vi "Scripting_ConvertNativeBaseClassToSubClass.vi"(0 "BaseClass":refnum<vi>, 1 "NewBaseClass":path=path "C:/Projects/P1G/N1_class/N1.lvclass", 5 "error in (no error)":errorcluster) -> (19 "error out":errorcluster={"status"=TRUE, "code"=1055, "source"="Property Node in Scripting_ConvertBaseClassToSubClass.vi"})   [LabVIEW 2020]
uses:
  <resource>/Framework/Providers/Open_GDS/ClassProviders/Provider_LvNativeClass/Templates/LvNativeTemplateNames.ctl
  <resource>/Framework/Providers/Open_GDS/ClassProviders/Provider_LvNativeClass/ClassWriterNative_class/ClassWriterNative.lvclass
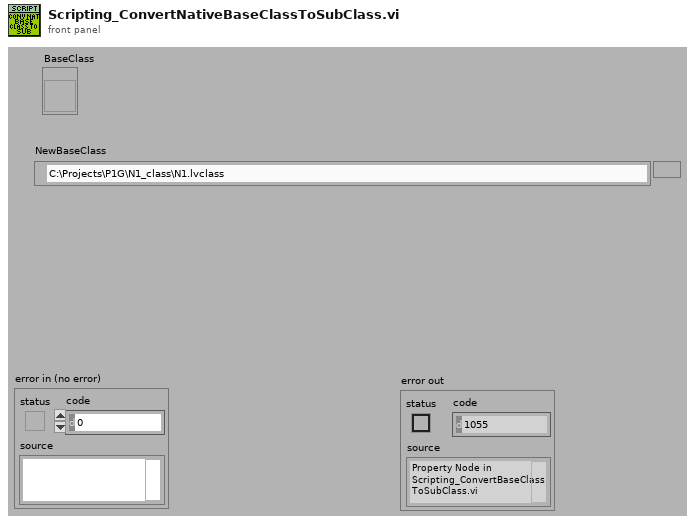
[diagram p1: front panel]
types:
  T1 = cluster{"NewBaseClass":refnum<vi>, "NewBaseCreate ":path, "NewBaseDestroy":path, " BaseClass":refnum<vi>, "BaseCreate ":path, "BaseDestroy":path, "BaseClassName":string, "AllBaseClassFiles":path[], "BaseNewVi":path, "BaseDeleteVi":path, "App":refnum<vi>}
  T2 = typedef "LvNativeTemplateNames.ctl" = enum16{"NativeBaseTemplate", "NativeSubTemplate", "NativeBaseTemplate_4x4x4", "NativeSubTemplate_4x4x4"}
  T3 = typedef "GDSLvCLass_ClassSettingsType.ctl" = cluster{"ClassProviderName":string, "ClassTemplateUsed":string, "ClassTemplateVersion":string, "ClassDescription":string, "PlugIns":T4[], "ConnectorPanePattern":string}
  T4 = typedef "GDSLvClass_PlugIn.ctl" = cluster{"Type":T5, "ID":string, "Version":string, "Path":path, "Name":string, "Data":variant}
  T5 = typedef "GDSLvClass_PlugInTypes.ctl" = enum16{"DesignPattern", "MethodTypes"}
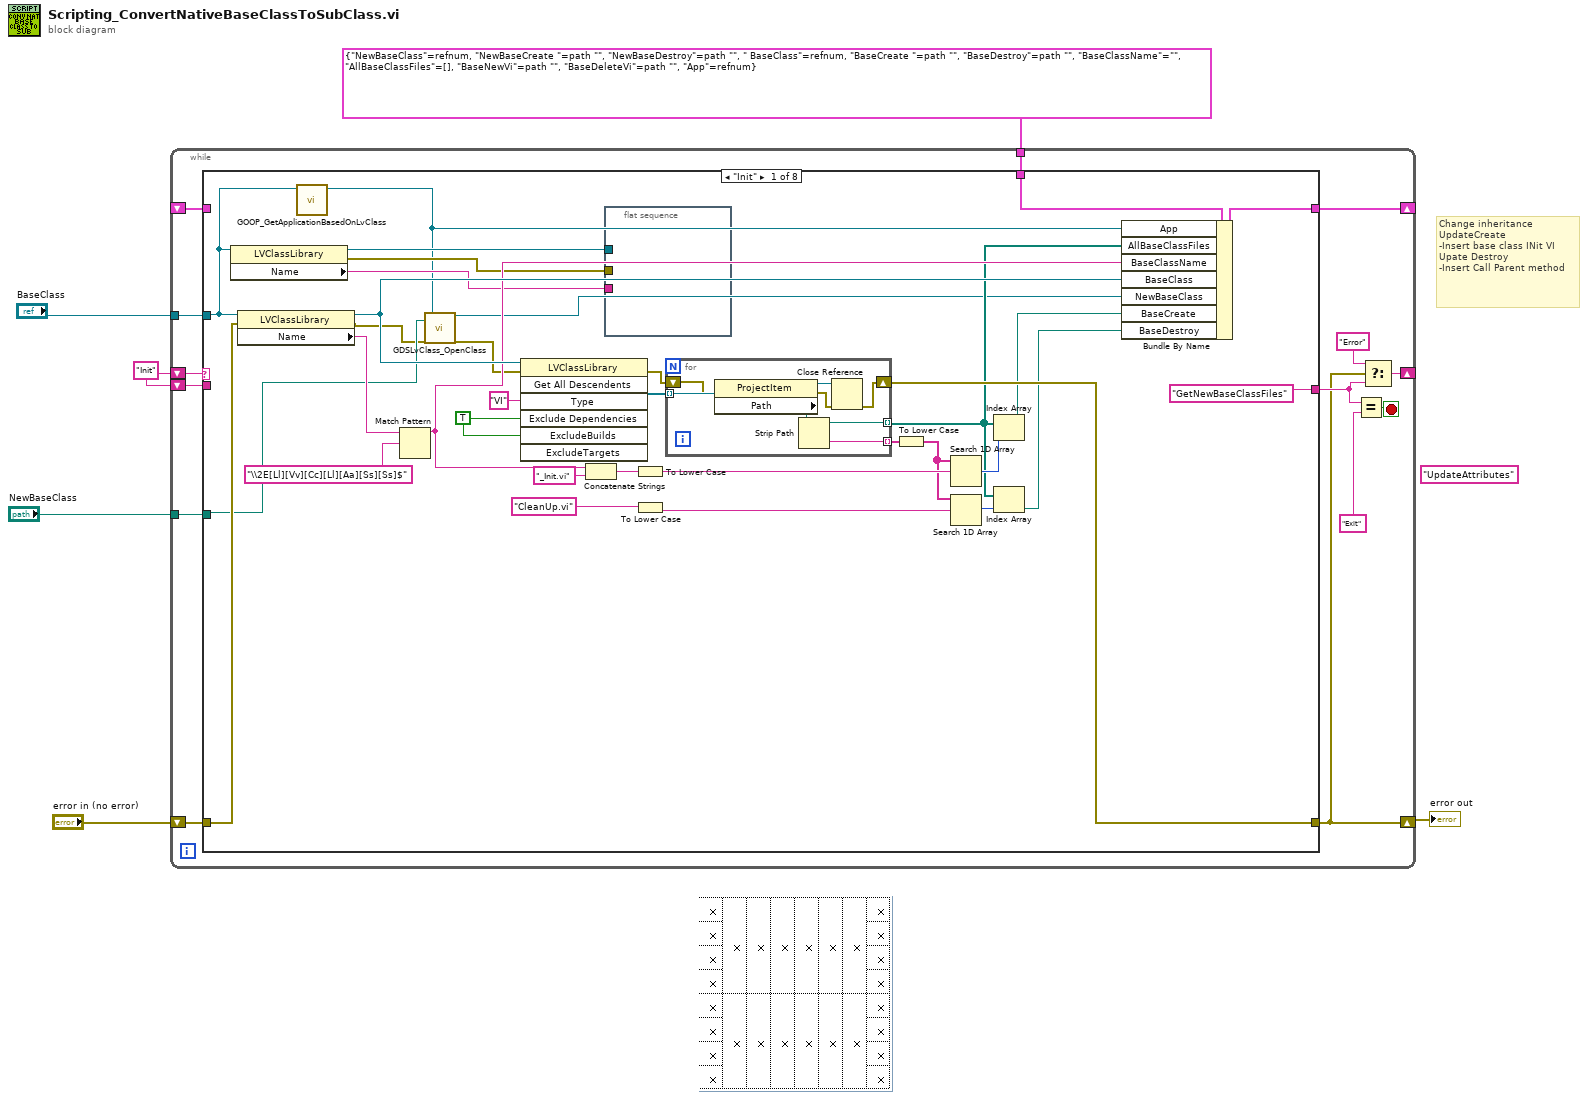
[diagram p0: block diagram]
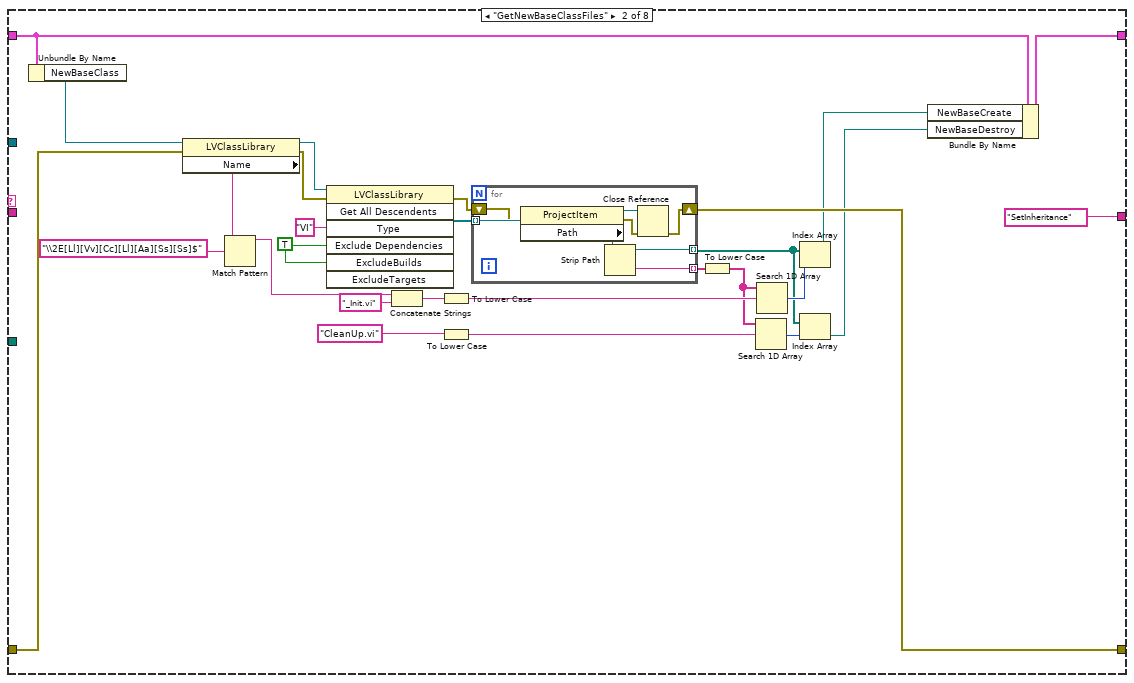
[diagram p2: hidden frame]
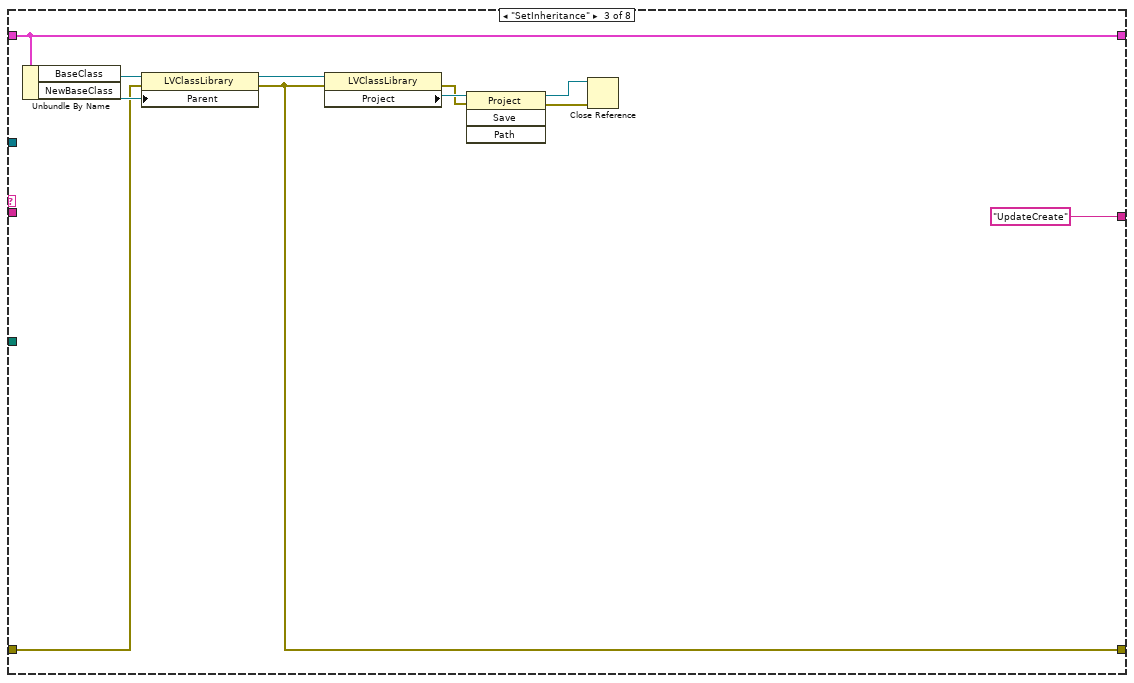
[diagram p3: hidden frame]
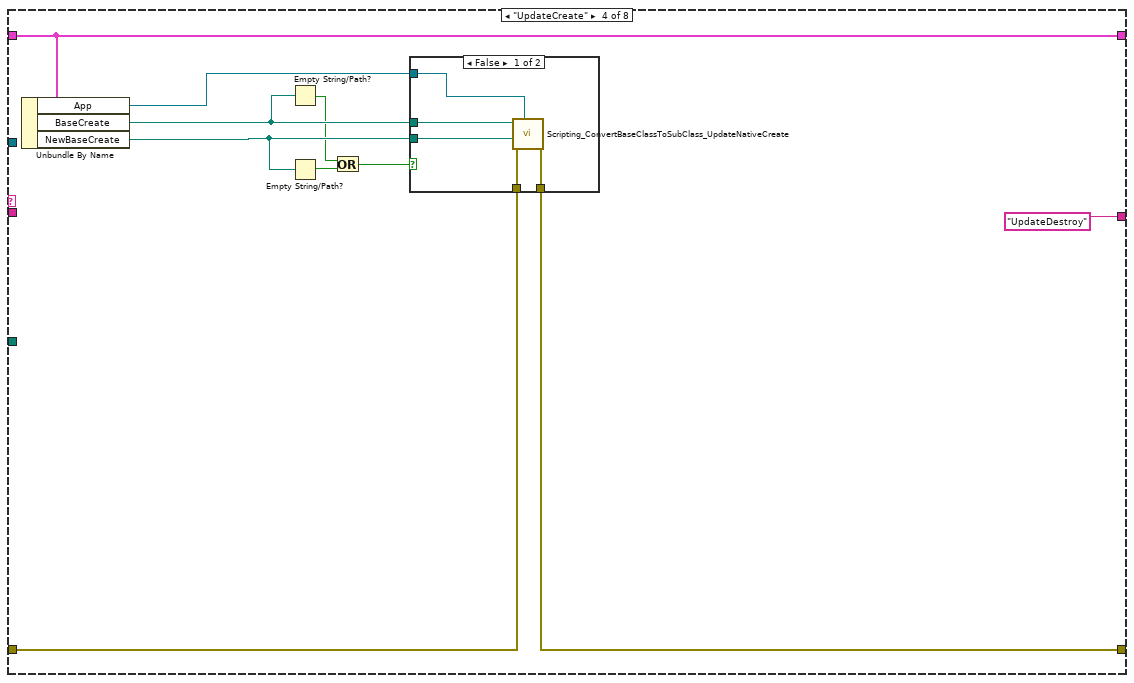
[diagram p4: hidden frame]
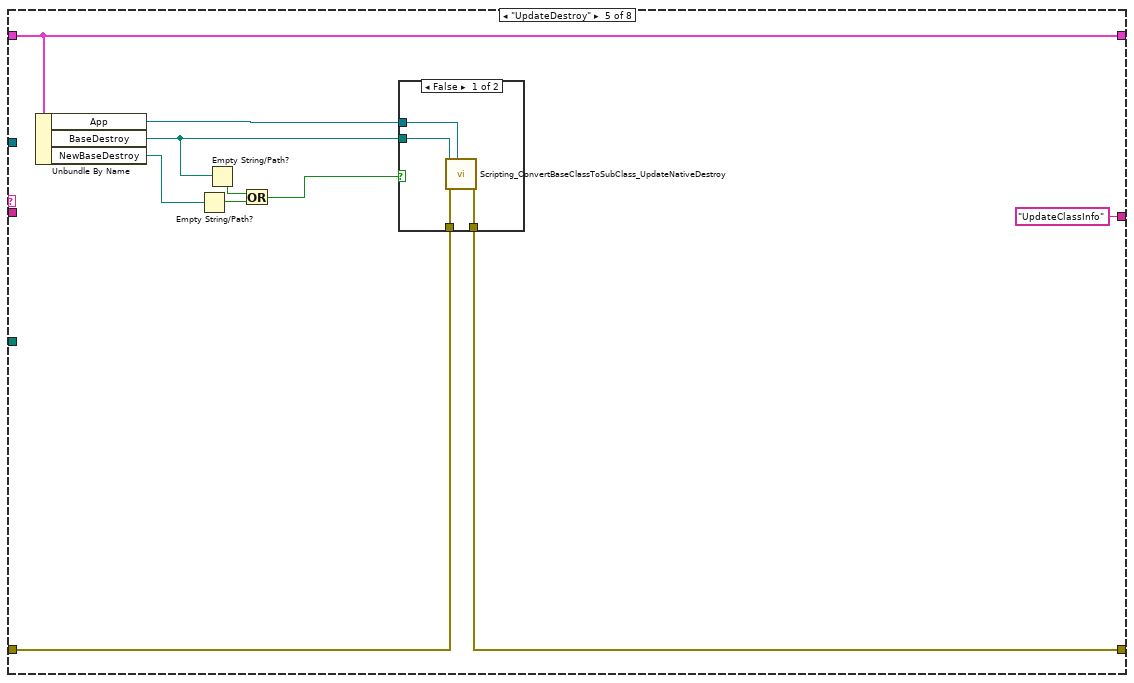
[diagram p6: hidden frame]
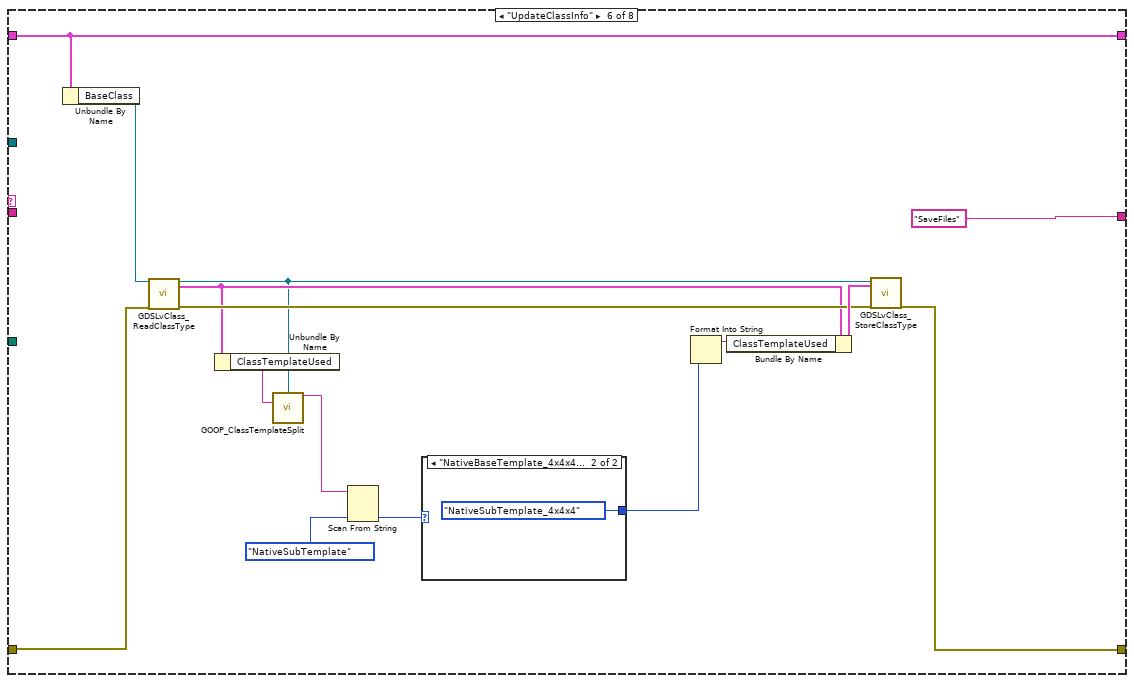
[diagram p8: hidden frame]
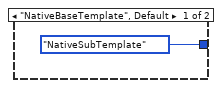
[diagram p9: hidden frame]
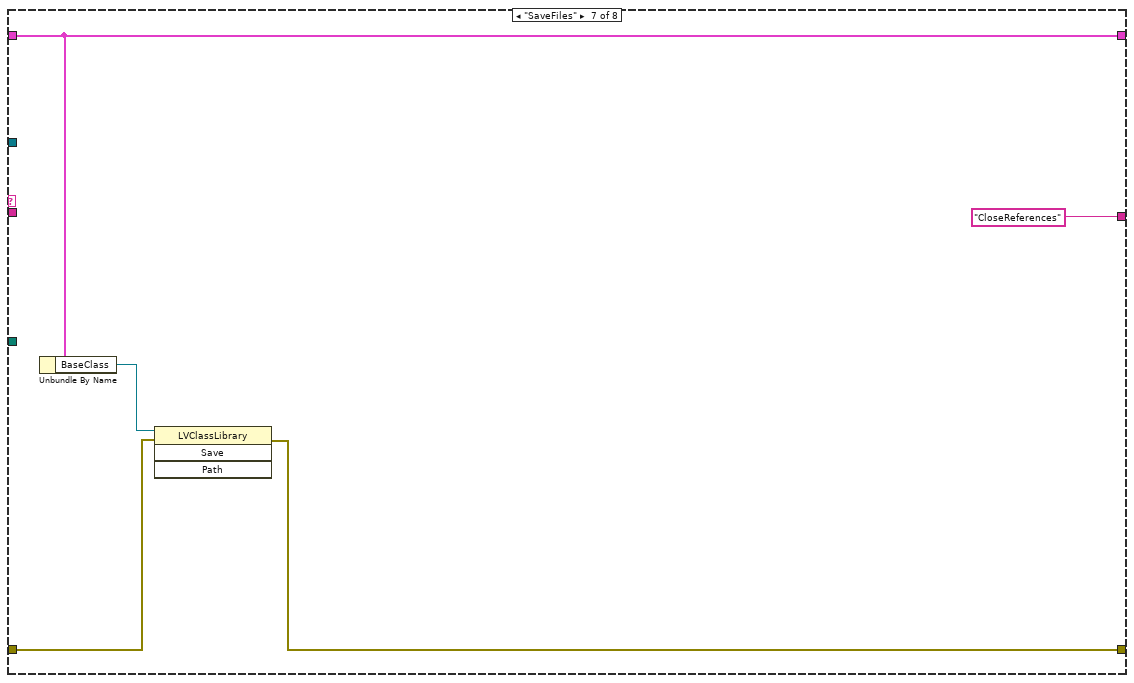
[diagram p10: hidden frame]
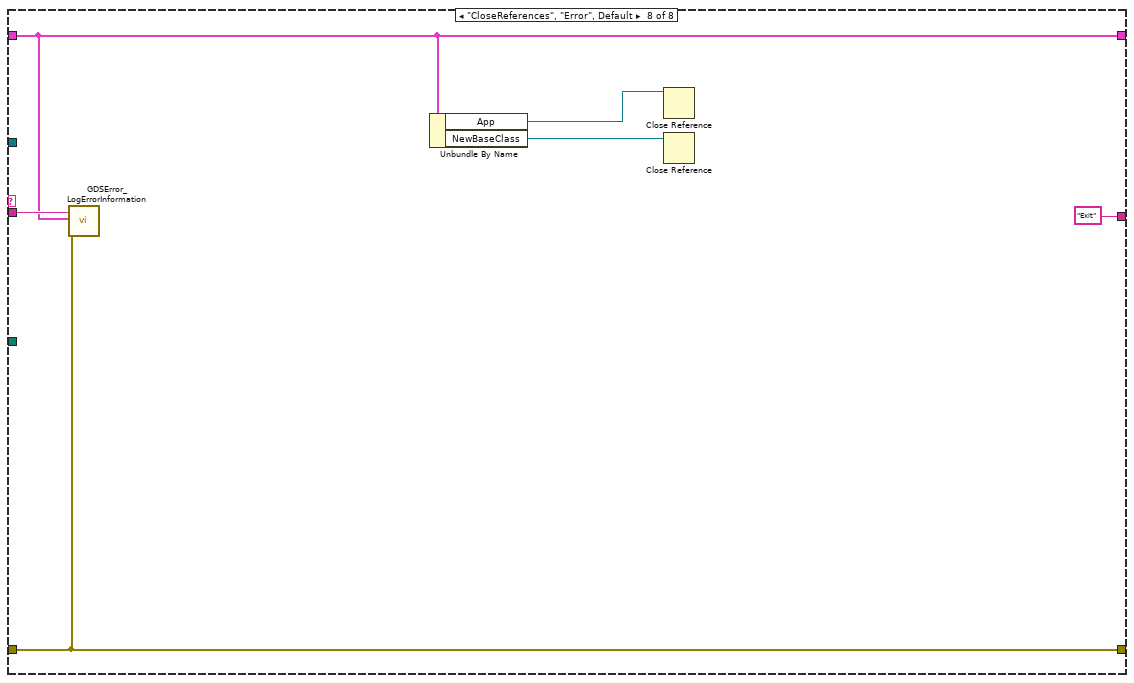
[diagram p11: hidden frame]
diagram:
  (unwired) "UpdateAttributes"
  w2 = "Init"
  # "Change inheritance\nUpdateCreate\n-Insert base class INit VI\nUpate Destroy\n-Insert Call Parent method"
  n1 = while {
    shift-right: [w13] -> w5
    shift-left: "error in (no error)" -> [w20]
    shift-right: [w18] -> _
    shift-left: w2 -> [w19]
    shift-right: [w12] -> _
    shift-left: _ -> [w11]
    tunnel: "BaseClass" -> [w10]
    tunnel: T1 {"NewBaseClass"=refnum, "NewBaseCreate "=path "", "NewBaseDestroy"=path "", " BaseClass"=refnum, "BaseCreate "=path "", "BaseDestroy"=path "", "BaseClassName"="", "AllBaseClassFiles"=[], "BaseNewVi"=path "", "BaseDeleteVi"=path "", "App"=refnum} -> [w9]
    tunnel: "NewBaseClass" -> [w8]
    shift-left: w2 -> [w7]
    stop <- w17 stop-if-true
    n2 = case shown="\"Init\"" w19 {
      tunnel: w20 -> [w38 w71 w103 w114 w130 w145 w156 w161]
      tunnel: [w44 w77 w96 w113 w129 w150 w155 w161] -> w13
      tunnel: ["GetNewBaseClassFiles" "SetInheritance" "UpdateCreate" "UpdateDestroy" "UpdateClassInfo" "SaveFiles" "CloseReferences" "Exit"] -> w14
      tunnel: [w53 w88 w105 w116 w132 w148 w159 w162] -> w12
      tunnel: w11 -> [_ w72 w105 w116 w132 w148 w159 w162]
      tunnel: w10 -> [w22 _ _ _ _ _ _ _]
      tunnel: w9 -> [w40 _ _ _ _ _ _ _]
      tunnel: w8 -> [w33 _ _ _ _ _ _ _]
      tunnel: w7 -> [_ _ _ _ _ _ _ w163]
      frame "Init" {
        w26 = TRUE ("ExcludeDependencies")
        n3 = property class="LVClassLibrary"(reference=w22) -> (reference out=w25:refnum<vi>, error out=w24:errorcluster, "Name"=w23:string)  [unwired: 1 in]
        n4 = property class="LVClassLibrary"(reference=w22, error in=w38) -> (reference out=w36:refnum<vi>, error out=w32:errorcluster, "Name"=w37:string)
        n5 = call <resource>:"GOOP_GetApplicationBasedOnLvClass.vi"("LVClassLibrary in"=w22) -> ("Application out"=w21:refnum<vi>)  [unwired: 9 in, 1 out]
        n6 = Match Pattern(string=w37, regular expression="\\2E[Ll][Vv][Cc][Ll][Aa][Ss][Ss]$") -> (before substring=w35:string)  [unwired: 1 in, 3 out]
        n7 = call <resource>:"GDSLvClass_OpenClass.vi"("ClassToOpen"=w33, "error in (no error)"=w32, "Project/ApplicationRef(If empty, currect active project will be used)"=w21) -> ("LVClass.Open"=w30:refnum<vi>, "error out"=w31:errorcluster)  [unwired: 15 in]
        n8 = invoke class="LVClassLibrary" method="Get All Descendents"(reference=w36, error in=w31, "Type"="VI", "Exclude Dependencies"=w26, "ExcludeBuilds"=w26) -> (error out=w50:errorcluster, "All Descendents"=w51:refnum<vi>[])  [unwired: 2 in, 5 out]
        n9 = Concatenate Strings(w35, "_Init.vi" ("string")) -> (w47:string)
        n10 = flat-sequence {
          tunnel: w25 -> [_]
          tunnel: w24 -> [_]
          tunnel: w23 -> [_]
          frame #0 {
          }
        }
        n11 = To Lower Case(string=w47) -> (all lower case string=w46:string)
        n12 = To Lower Case(string="CleanUp.vi") -> (all lower case string=w27:string)
        n13 = for {
          tunnel: w51 -> [w61] mode=indexing
          shift-right: [w57] -> w44
          shift-left: w50 -> [w58]
          tunnel: [w56] -> w34 mode=indexing
          tunnel: [w55] -> w48 mode=indexing
          n14 = property class="ProjectItem"(reference=w61, error in=w58) -> (reference out=w60:refnum<vi>, error out=w59:errorcluster, "Path"=w56:path)
          n15 = Strip Path(path=w56) -> (name=w55:string)  [unwired: 1 out]
          n16 = Close Reference(reference=w60, error in (no error)=w59) -> (error out=w57:errorcluster)
        }
        n17 = To Lower Case(string=w48) -> (all lower case string=w28:string[])
        n18 = Search 1D Array(1D array=w28, element=w46) -> (index of element=w45:i32)  [unwired: 1 in]
        n19 = Search 1D Array(1D array=w28, element=w27) -> (index of element=w29:i32)  [unwired: 1 in]
        n20 = Index Array(array=w34, index=w45) -> (element=w42:path)
        n21 = Index Array(array=w34, index=w29) -> (element=w41:path)
        n22 = Bundle By Name(cluster=w40, "App"=w21, "AllBaseClassFiles"=w34, "BaseClassName"=w35, "BaseClass"=w36, "NewBaseClass"=w30, "BaseCreate"=w42, "BaseDestroy"=w41) -> (w53:T1)
      }
      frame "GetNewBaseClassFiles" {
        w62 = TRUE ("ExcludeDependencies")
        n23 = Unbundle By Name(w72) -> ("NewBaseClass"=w69:refnum<vi>)
        n24 = property class="LVClassLibrary"(reference=w69, error in=w71) -> (reference out=w83:refnum<vi>, error out=w84:errorcluster, "Name"=w70:string)
        n25 = Match Pattern(string=w70, regular expression="\\2E[Ll][Vv][Cc][Ll][Aa][Ss][Ss]$") -> (before substring=w65:string)  [unwired: 1 in, 3 out]
        n26 = invoke class="LVClassLibrary" method="Get All Descendents"(reference=w83, error in=w84, "Type"="VI", "Exclude Dependencies"=w62, "ExcludeBuilds"=w62) -> (error out=w85:errorcluster, "All Descendents"=w86:refnum<vi>[])  [unwired: 2 in, 5 out]
        n27 = Concatenate Strings(w65, "_Init.vi" ("string")) -> (w80:string)
        n28 = To Lower Case(string=w80) -> (all lower case string=w79:string)
        n29 = To Lower Case(string="CleanUp.vi") -> (all lower case string=w75:string)
        n30 = for {
          tunnel: w86 -> [w95] mode=indexing
          shift-right: [w91] -> w77
          shift-left: w85 -> [w92]
          tunnel: [w90] -> w67 mode=indexing
          tunnel: [w89] -> w81 mode=indexing
          n31 = property class="ProjectItem"(reference=w95, error in=w92) -> (reference out=w94:refnum<vi>, error out=w93:errorcluster, "Path"=w90:path)
          n32 = Strip Path(path=w90) -> (name=w89:string)  [unwired: 1 out]
          n33 = Close Reference(reference=w94, error in (no error)=w93) -> (error out=w91:errorcluster)
        }
        n34 = To Lower Case(string=w81) -> (all lower case string=w66:string[])
        n35 = Search 1D Array(1D array=w66, element=w75) -> (index of element=w63:i32)  [unwired: 1 in]
        n36 = Search 1D Array(1D array=w66, element=w79) -> (index of element=w78:i32)  [unwired: 1 in]
        n37 = Index Array(array=w67, index=w78) -> (element=w74:path)
        n38 = Index Array(array=w67, index=w63) -> (element=w73:path)
        n39 = Bundle By Name(cluster=w72, "NewBaseCreate"=w74, "NewBaseDestroy"=w73) -> (w88:T1)
      }
      frame "SetInheritance" {
        n40 = Unbundle By Name(w105) -> ("BaseClass"=w106:refnum<vi>, "NewBaseClass"=w104:refnum<vi>)
        n41 = property class="LVClassLibrary"(reference=w106, error in=w103, "Parent"=w104) -> (reference out=w101:refnum<vi>, error out=w96:errorcluster)
        n42 = property class="LVClassLibrary"(reference=w101, error in=w96) -> (error out=w97:errorcluster, "Project"=w100:refnum<vi>)  [unwired: 1 out]
        n43 = invoke class="Project" method="Save"(reference=w100, error in=w97) -> (reference out=w98:refnum<vi>, error out=w99:errorcluster)  [unwired: 2 in, 2 out]
        n44 = Close Reference(reference=w98, error in (no error)=w99) -> ()  [unwired: 1 out]
      }
      frame "UpdateCreate" {
        n45 = Unbundle By Name(w116) -> ("App"=w111:refnum<vi>, "BaseCreate"=w112:path, "NewBaseCreate"=w110:path)
        n46 = Empty String/Path?(string/path=w112) -> (empty?=w108:bool)
        n47 = Empty String/Path?(string/path=w110) -> (empty?=w109:bool)
        n48 = Or(x=w108, y=w109) -> (x .or. y?=w107:bool)
        n49 = case shown="False" w107 {
          tunnel: w112 -> [w121 _]
          tunnel: w114 -> [w120 w122]
          tunnel: [w119 w122] -> w113
          tunnel: w110 -> [w118 _]
          tunnel: w111 -> [w117 _]
          frame False {
            n50 = call <resource>:"Scripting_ConvertBaseClassToSubClass_UpdateNativeCreate.vi"("AppRef"=w117, "error in (no error)"=w120, "NewBaseClassInitViPath"=w118, "CurrentBaseInitVI"=w121) -> ("error out"=w119:errorcluster)  [unwired: 7 in]
          }
          frame True {
          }
        }
      }
      frame "UpdateDestroy" {
        n51 = Unbundle By Name(w132) -> ("App"=w127:refnum<vi>, "BaseDestroy"=w128:path, "NewBaseDestroy"=w125:path)
        n52 = Empty String/Path?(string/path=w125) -> (empty?=w126:bool)
        n53 = Empty String/Path?(string/path=w128) -> (empty?=w124:bool)
        n54 = Or(x=w124, y=w126) -> (x .or. y?=w123:bool)
        n55 = case shown="False" w123 {
          tunnel: w130 -> [w136 w137]
          tunnel: [w135 w137] -> w129
          tunnel: w128 -> [w134 _]
          tunnel: w127 -> [w133 _]
          frame False {
            n56 = call <resource>:"Scripting_ConvertBaseClassToSubClass_UpdateNativeDestroy.vi"("AppRef"=w133, "error in (no error)"=w136, "CurrentBaseCleanUpVI"=w134) -> ("error out"=w135:errorcluster)  [unwired: 8 in]
          }
          frame True {
          }
        }
      }
      frame "UpdateClassInfo" {
        n57 = Unbundle By Name(w148) -> ("BaseClass"=w146:refnum<vi>)
        n58 = call <resource>:"GDSLvClass_ReadClassType.vi"("Class Refnum In"=w146, "error in (no error)"=w145) -> ("Class Refnum Out"=w138:refnum<vi>, "ClassSettings"=w144:T3, "error out"=w147:errorcluster)  [unwired: 15 in]
        n59 = Unbundle By Name(w144) -> ("ClassTemplateUsed"=w140:string)
        n60 = call <resource>:"GOOP_ClassTemplateSplit.vi"("ClassItemRefIn"=w138, "FullClassTemplate"=w140) -> ("StandardTemplate"=w139:string)  [unwired: 12 in, 1 out]
        n61 = Scan From String(input string=w139, default 1=LvNativeTemplateNames."NativeSubTemplate" ("TemplateNames")) -> (output 1=w142:T2)  [unwired: 3 in, 3 out]
        n62 = case shown="\"NativeBaseTemplate_4x4x4\"" w142 {
          tunnel: [LvNativeTemplateNames."NativeSubTemplate" ("TemplateNames") LvNativeTemplateNames."NativeSubTemplate_4x4x4" ("TemplateNames")] -> w141
          frame "NativeBaseTemplate", Default {
          }
          frame "NativeBaseTemplate_4x4x4" {
          }
        }
        n63 = Format Into String(w141) -> (resulting string=w151:string)  [unwired: 3 in, 1 out]
        n64 = Bundle By Name(cluster=w144, "ClassTemplateUsed"=w151) -> (w152:T3)
        n65 = call <resource>:"GDSLvClass_StoreClassType.vi"("Class Refnum In"=w138, "ClassSettings"=w152, "error in (no error)"=w147) -> ("error out"=w150:errorcluster)  [unwired: 15 in, 1 out]
      }
      frame "SaveFiles" {
        n66 = Unbundle By Name(w159) -> ("BaseClass"=w158:refnum<vi>)
        n67 = invoke class="LVClassLibrary" method="Save"(reference=w158, error in=w156) -> (error out=w155:errorcluster)  [unwired: 2 in, 3 out]
      }
      frame "CloseReferences", "Error", Default {
        n68 = call <resource>:"GDSError_LogErrorInformation.vi"("State"=w163, "LocalVariableData"=w162, "error in (no error)"=w161) -> ()  [unwired: 16 in, 1 out]
        n69 = Unbundle By Name(w162) -> ("App"=w160:refnum<vi>, "NewBaseClass"=w165:refnum<vi>)
        n70 = Close Reference(reference=w160) -> ()  [unwired: 1 in, 1 out]
        n71 = Close Reference(reference=w165) -> ()  [unwired: 1 in, 1 out]
      }
    }
    n72 = Equal?(x=w14, y="Exit") -> (x = y?=w17:bool)
    n73 = Select(t="Error", s=w13, f=w14) -> (s? t:f=w18:string)
  }
  "error out" <- w5
